vi "Init TCP.vi"(8 "error in (no error)":errorcluster, 10 "Port":u16=80, 11 "Server in":refnum<class "Server.lvclass">) -> (0 "error out":errorcluster, 3 "Server out":refnum<class "Server.lvclass">)   [LabVIEW 2020, in "HTTP Server.lvlib" / "Server.lvclass"]
uses:
  Server.lvclass
  Server.lvclass/Server.ctl
  Insecure Connection Callback.vi
  HTTP TCP Server/HTTP TCP Server.lvclass
  lv-stream/stream/Endpoint/Endpoint.lvclass
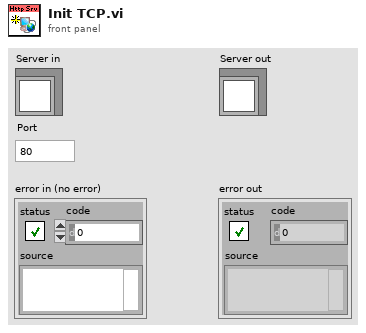
[diagram p1: front panel]
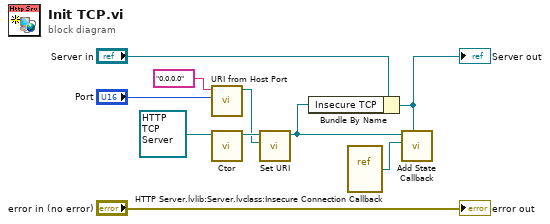
[diagram p0: block diagram]
diagram:
  n1 = call "URI from Host Port.vi"("Port"="Port", "Host"="0.0.0.0") -> ("URI"=w6:refnum<class "URI.lvclass">)  [unwired: 9 in]
  n2 = call-dynamic "Ctor.vi"("TCP Server in"=refnum<class "HTTP TCP Server.lvclass"> refnum ("HTTP Server.lvlib:HTTP TCP Server")) -> ("TCP Server out"=w7:refnum<class "HTTP TCP Server.lvclass">)  [unwired: 9 in, 1 out]
  n3 = call "Set URI.vi"("URI"=w6, "Endpoint in"=w7) -> ("Endpoint out"=w4:refnum<class "Endpoint.lvclass">)  [unwired: 8 in, 1 out]
  n4 = Bundle By Name(cluster="Server in", "Insecure TCP"=w4) -> (w3:refnum<class "Server.lvclass">)
  "Server out" <- w3
  n5 = vi-ref "HTTP Server.lvlib:Server.lvclass:Insecure Connection Callback.vi"() -> (w2:refnum<vi>)
  n6 = call-dynamic "Add State Callback.vi"("Owner (None)"=w3, "Callback"=w2, "Endpoint in"=w4) -> ()  [unwired: 7 in, 2 out]
  "error out" <- "error in (no error)"
